vi "Destroy.vi"(8 "error in (no error)":errorcluster, 11 "EventTestListener in":refnum<class "EventTestListener.lvclass">) -> (0 "error out":errorcluster)   [LabVIEW 2019, in "TestExplorer.lvlib" / "EventTestListener.lvclass"]
uses:
  EventTestListener.lvclass
  EventTestListener.lvclass/EventTestListener.ctl
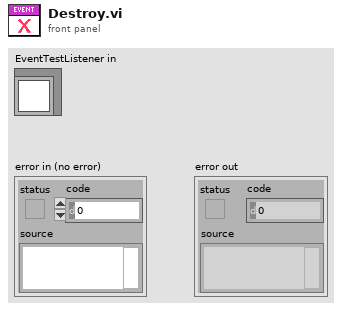
[diagram p1: front panel]
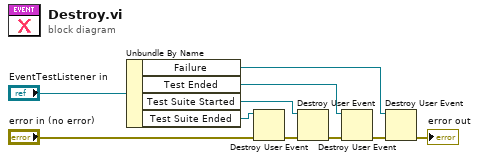
[diagram p0: block diagram]
diagram:
  n1 = Unbundle By Name("EventTestListener in") -> ("Failure"=w8:refnum<user-event>, "Test Ended"=w6:refnum<user-event>, "Test Suite Started"=w4:refnum<user-event>, "Test Suite Ended"=w1:refnum<user-event>)
  n2 = Destroy User Event(user event=w1, error in="error in (no error)") -> (error out=w2:errorcluster)
  n3 = Destroy User Event(user event=w4, error in=w2) -> (error out=w5:errorcluster)
  n4 = Destroy User Event(user event=w6, error in=w5) -> (error out=w7:errorcluster)
  n5 = Destroy User Event(user event=w8, error in=w7) -> (error out=→"error out":errorcluster)
